vi "GOOP_Provider_GetTranslatedName.vi"(11 "ProviderName":string) -> (3 "TranslatedName":string)   [LabVIEW 2020]
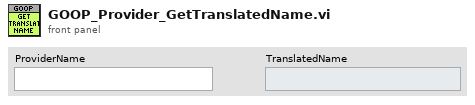
[diagram p1: front panel]
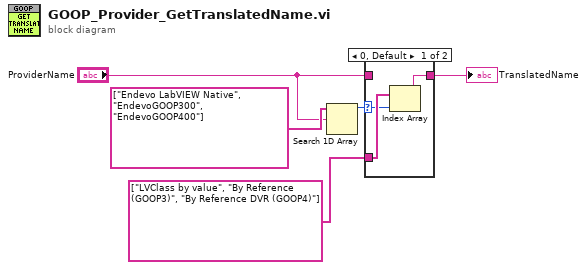
[diagram p0: block diagram]
diagram:
  n1 = Search 1D Array(1D array=string[] ["Endevo LabVIEW Native", "EndevoGOOP300", "EndevoGOOP400"] ("AllClassProviders"), element="ProviderName") -> (index of element=w1:i32)  [unwired: 1 in]
  n2 = case shown="0, Default" w1 {
    selector: w1 -> [w7 _]
    tunnel: "ProviderName" -> [_ w9]
    tunnel: [w6 w9] -> w3
    tunnel: string[] ["LVClass by value", "By Reference (GOOP3)", "By Reference DVR (GOOP4)"] ("AllClassProviders") -> [w8 _]
    frame 0, Default {
      n3 = Index Array(array=w8, index=w7) -> (element=w6:string)
    }
    frame -1 {
    }
  }
  "TranslatedName" <- w3
